vi "ClassPanel.vi"(8 "error in (no error)":errorcluster caption="entrée d'erreur (pas d'erreur)", 11 "EG_G5210.lvclass":refnum<class "EGG5210.lvclass">) -> (0 "error out":errorcluster caption="sortie d'erreur", 3 "EG_G5210.lvclass Out":refnum<class "EGG5210.lvclass">)   [LabVIEW 2012, in "EGG5210.lvclass"]
uses:
  EGG5210.lvclass
panel:
  in  "Acq":bool
  out "Sensitivity":u16(ring)=13 items=["100 nV", "300 nV", "1 µV", "3 µV", "10 µV", "30 µV", "100µV", "300 µV", "1 mV", "3 mV", "10 mV", "30 mV", "100 mV", "300 mV", "1 V", "3 V"]
  out "Phase":dbl=1000.0 caption="Phase (°)" min=0.0 step=0.1 format="%#.1f"
  out "MAG":dbl=1000.0 caption="MAG (V)" min=0.0 step=0.1 format="%#.1f"
  out "UNLCK":bool caption="SpexMov"
  out "X":dbl=1000.0 caption="X (V)" min=0.0 step=0.1 format="%#.1f"
  in  "Stop":bool
  out "Init Program":bool
  out "OVLD":bool caption="SpexMov"
  in  "Update":bool caption="stopSpectro"
  out "Y":dbl=1000.0 caption="Y (V)" min=0.0 step=0.1 format="%#.1f"
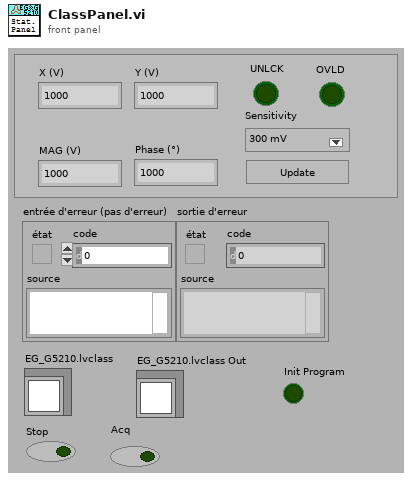
[diagram p1: front panel]
types:
  T1 = enum8{"Enabled", "Disabled", "Disabled and Grayed Out"}
  T2 = enum16{"X Output", "Y Output", "X and Y Output", "Mag", "Phase", "Mag & Phase", "X,Y,Mag & Phase", "Noise", "Aux In 1", "Aux In 2", "Aux In 3", "Aux In 4"}
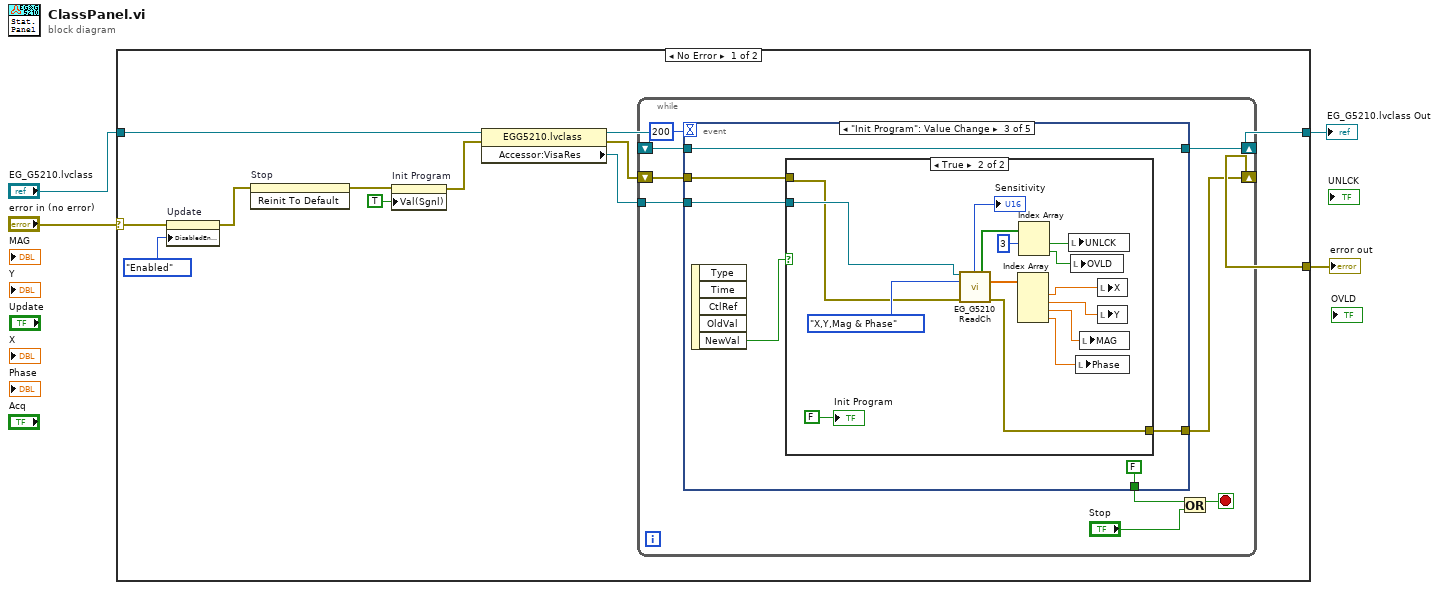
[diagram p0: block diagram]
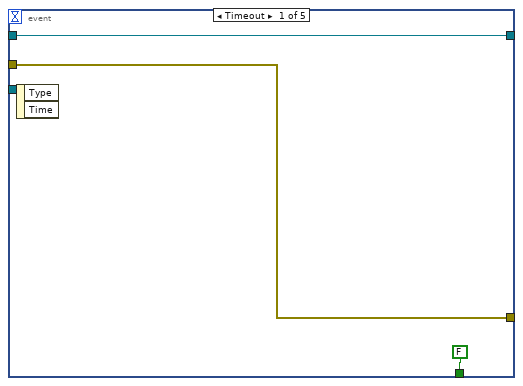
[diagram p2: hidden frame]
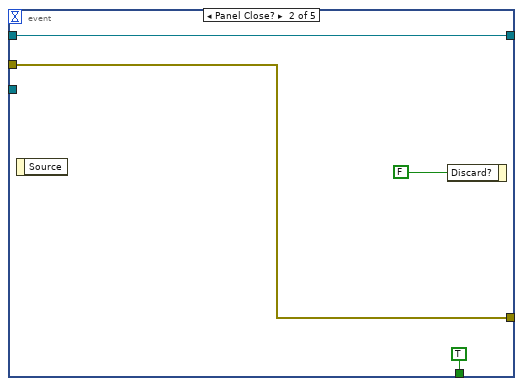
[diagram p3: hidden frame]
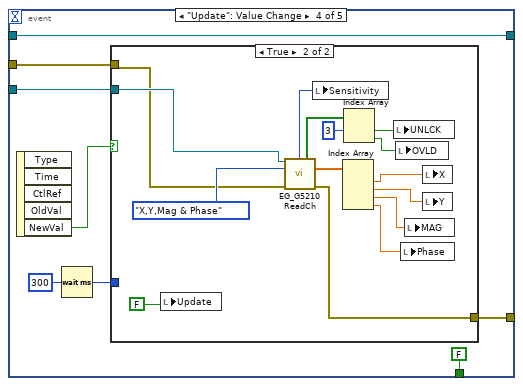
[diagram p5: hidden frame]
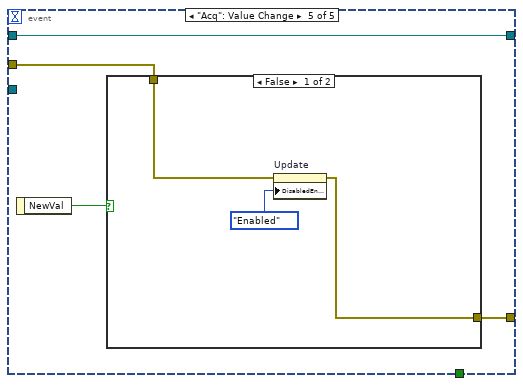
[diagram p7: hidden frame]
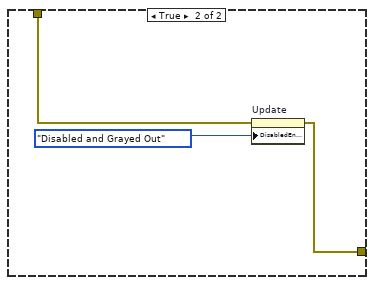
[diagram p8: hidden frame]
diagram:
  n1 = case shown="No Error" "error in (no error)" {
    selector: "error in (no error)" -> [w6 w90]
    tunnel: [w16 w90] -> w3
    tunnel: "EG_G5210.lvclass" -> [w15 w89]
    tunnel: [w12 w89] -> w1
    frame No Error {
      n2 = property on="Update" class="Bool (strict)"(error in=w6, "DisabledEnum"=T1."Enabled" ("Désactivé")) -> (error out=w5:errorcluster)  [unwired: 1 in, 1 out]
      n3 = invoke on="Stop" class="Bool (strict)" method="Reinit To Default"(error in=w5) -> (error out=w11:errorcluster)  [unwired: 2 in, 2 out]
      n4 = property on="Init Program" class="Bool (strict)"(error in=w11, "Val(Sgnl)"=TRUE ("Valeur (Signalisation)")) -> (error out=w10:errorcluster)  [unwired: 1 in, 1 out]
      n5 = property class="EGG5210.lvclass"(reference=w15, error in=w10) -> (reference out=w14:refnum<class "EGG5210.lvclass">, error out=w8:errorcluster, "Accessor:VisaRes"=w9:refnum<visa-resource-name>)
      n6 = while {
        shift-right: [w23] -> w16
        shift-left: w8 -> [w24]
        tunnel: w9 -> [w20]
        shift-right: [w19] -> w12
        shift-left: w14 -> [w22]
        stop <- w18 stop-if-true
        n7 = event shown="[2] \"Init Program\": Value Change" {
          selector: _ -> [_ _ _ _ _]
          dyn-events: _ -> [_ _ _ _ _]
          timeout: 200 -> [_ _ _ _ _]
          tunnel: w24 -> [w26 w30 w36 w61 w82]
          tunnel: [w26 w30 w35 w60 w80] -> w23
          tunnel: w22 -> [w27 w29 w34 w59 w79]
          tunnel: [FALSE TRUE FALSE FALSE _] -> w21
          tunnel: [w27 w29 w34 w59 w79] -> w19
          tunnel: w20 -> [_ _ w37 w62 _]
          event Timeout {
            n8 = event-data() -> ()  [unwired: 1 in, 2 out]
          }
          event Panel Close? {
            n9 = event-data() -> ()  [unwired: 1 in, 1 out]
            n10 = event-data("Discard?"=FALSE ("Rejeter ?")) -> ()  [unwired: 1 in, 1 out]
          }
          event "Init Program": Value Change {
            n11 = event-data() -> ("NewVal"=w38:bool)  [unwired: 1 in, 4 out]
            n12 = case shown="True" w38 {
              tunnel: w37 -> [_ w53]
              tunnel: w36 -> [w39 w48]
              tunnel: [w39 w50] -> w35
              frame False {
              }
              frame True {
                n13 = call <userlib>:"EG_G5210 ReadCh.vi"("VISA Rsrc"=w53, "Channel"=T2."X,Y,Mag & Phase", "error in (no error)"=w48) -> ("Sensitivity"=→"Sensitivity":u16, "Status Byte"=w47:bool[], "Outputs"=w49:dbl[], "error out"=w50:errorcluster)  [unwired: 5 in, 4 out]
                n14 = Index Array(array=w49) -> (element #1=w43:dbl, element #2=w42:dbl, element #3=w41:dbl, element #4=w40:dbl)  [unwired: 4 in]
                n15 = Index Array(array=w47, index #1=3 ("indice")) -> (element #1=w45:bool, element #2=w44:bool)  [unwired: 1 in]
                n16 = local write "UNLCK"(w45) -> ()
                n17 = local write "OVLD"(w44) -> ()
                n18 = local write "Phase"(w40) -> ()
                n19 = local write "MAG"(w41) -> ()
                n20 = local write "X"(w43) -> ()
                n21 = local write "Y"(w42) -> ()
                "Init Program" <- FALSE
              }
            }
          }
          event "Update": Value Change {
            n22 = event-data() -> ("NewVal"=w57:bool)  [unwired: 1 in, 4 out]
            n23 = Wait (ms)(milliseconds to wait=u32 300 ("attente (ms)")) -> (millisecond timer value=w56:u32)
            n24 = case shown="True" w57 {
              tunnel: w62 -> [_ w78]
              tunnel: w61 -> [w63 w74]
              tunnel: [w63 w76] -> w60
              tunnel: w56 -> [_ _]
              frame False {
              }
              frame True {
                n25 = local write "Update"(FALSE) -> ()
                n26 = call <userlib>:"EG_G5210 ReadCh.vi"("VISA Rsrc"=w78, "Channel"=T2."X,Y,Mag & Phase", "error in (no error)"=w74) -> ("Sensitivity"=w65:u16, "Status Byte"=w73:bool[], "Outputs"=w75:dbl[], "error out"=w76:errorcluster)  [unwired: 5 in, 4 out]
                n27 = local write "Sensitivity"(w65) -> ()
                n28 = Index Array(array=w75) -> (element #1=w69:dbl, element #2=w68:dbl, element #3=w67:dbl, element #4=w66:dbl)  [unwired: 4 in]
                n29 = Index Array(array=w73, index #1=3 ("indice")) -> (element #1=w71:bool, element #2=w70:bool)  [unwired: 1 in]
                n30 = local write "UNLCK"(w71) -> ()
                n31 = local write "OVLD"(w70) -> ()
                n32 = local write "Phase"(w66) -> ()
                n33 = local write "MAG"(w67) -> ()
                n34 = local write "X"(w69) -> ()
                n35 = local write "Y"(w68) -> ()
              }
            }
          }
          event "Acq": Value Change {
            n36 = event-data() -> ("NewVal"=w81:bool)  [unwired: 1 in]
            n37 = case shown="False" w81 {
              tunnel: w82 -> [w84 w87]
              tunnel: [w83 w86] -> w80
              frame False {
                n38 = property on="Update" class="Bool (strict)"(error in=w84, "DisabledEnum"=T1."Enabled" ("Désactivé")) -> (error out=w83:errorcluster)  [unwired: 1 in, 1 out]
              }
              frame True {
                n39 = property on="Update" class="Bool (strict)"(error in=w87, "DisabledEnum"=T1."Disabled and Grayed Out" ("Désactivé")) -> (error out=w86:errorcluster)  [unwired: 1 in, 1 out]
              }
            }
          }
        }
        n40 = Or(x=w21, y="Stop") -> (x .or. y?=w18:bool)
      }
    }
    frame Error {
    }
  }
  "error out" <- w3
  "EG_G5210.lvclass Out" <- w1
